vi "Differential_Yuhe.vi"(8 "dy/dx vs x":bool=TRUE, 9 "step":dbl=5.0, 10 "dv":dbl=5.0, 11 "A vs B":cluster{dbl[], dbl[]}[](graph)) -> (3 "A vs B 2":cluster{dbl[], dbl[]}[](graph))   [LabVIEW 2020]
uses:
  <vilib>/Analysis/baseanly.llb/Mean (DBL).vi
  <vilib>/Analysis/NI_AALPro.lvlib
  <vilib>/Analysis/NI_AALBase.lvlib
panel:
  in  "parameter bounds":T1={"amp min"=-inf, "amp max"=inf, "power min"=-inf, "power max"=inf, "offset min"=0.0, "offset max"=0.0}
  out "residue":dbl
  out "amplitude":dbl
  out "Fitoffset":dbl
  out "power":dbl
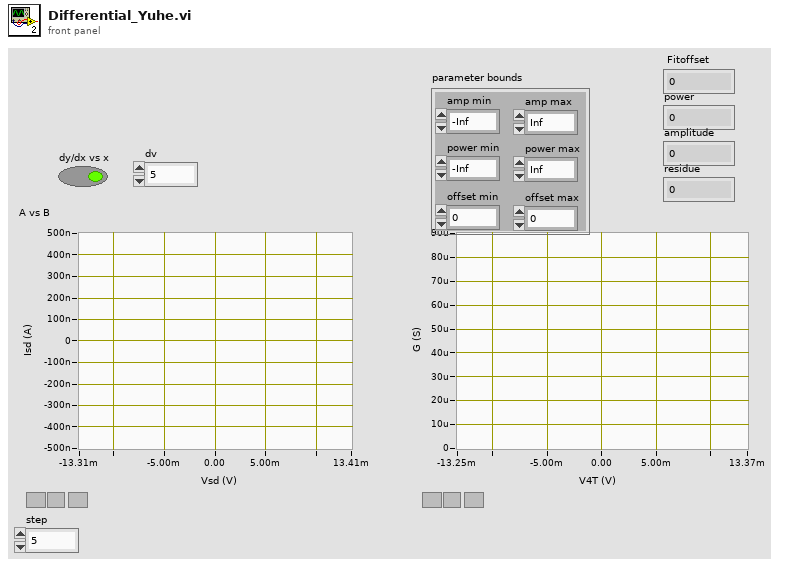
[diagram p1: front panel]
types:
  T1 = cluster{"amp min":dbl, "amp max":dbl, "power min":dbl, "power max":dbl, "offset min":dbl, "offset max":dbl}
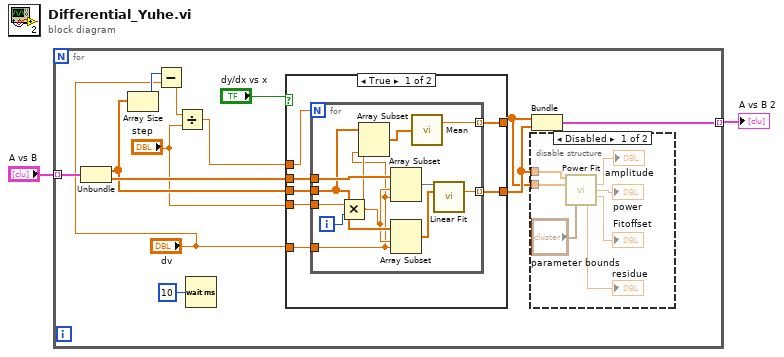
[diagram p0: block diagram]
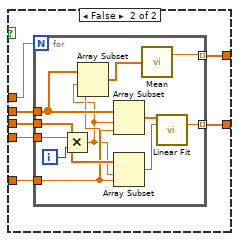
[diagram p3: hidden frame]
diagram:
  n1 = for {
    tunnel: "A vs B" -> [w13] mode=indexing
    tunnel: [w12] -> w1 mode=indexing
    n2 = Unbundle(w13) -> (w11:dbl[], w15:dbl[])
    n3 = Array Size(array=w11) -> (size(s)=w8:i32)
    n4 = Subtract(x=w8, y="dv") -> (x-y=w6:dbl)
    n5 = Divide(x=w6, y="step") -> (x/y=w10:dbl)
    n6 = Wait (ms)(milliseconds to wait=u32 10) -> ()  [unwired: 1 out]
    n7 = case shown="True" "dy/dx vs x" {
      tunnel: w10 -> [w29 w47]
      tunnel: "dv" -> [w28 w46]
      tunnel: [w27 w45] -> w4
      tunnel: w11 -> [w25 w43]
      tunnel: w15 -> [w26 w44]
      tunnel: [w23 w41] -> w3
      tunnel: "step" -> [w24 w42]
      frame True {
        n8 = for {
          N: w29 -> [_]
          tunnel: w25 -> [w34]
          tunnel: w26 -> [w40]
          tunnel: w28 -> [w32]
          tunnel: [w39] -> w27 mode=indexing
          tunnel: w24 -> [w38]
          tunnel: [w30] -> w23 mode=indexing
          i -> [w37]
          n9 = Multiply(x=w38, y=w37) -> (x*y=w33:dbl)
          n10 = Array Subset(array=w34, index=w33, length=w32) -> (w31:dbl[])
          n11 = Array Subset(array=w40, index=w33, length=w32) -> (w36:dbl[])
          n12 = Array Subset(array=w34, index=w33, length=w32) -> (w35:dbl[])
          n13 = call-poly <vilib>:"Mean.vi"("X"=w31) -> ("mean"=w30:dbl)  [unwired: 1 out]
          n14 = call <vilib>:"Linear Fit.vi"("Y"=w36, "X"=w35) -> ("slope"=w39:dbl)  [unwired: 9 in, 4 out]
        }
      }
      frame False {
        n15 = for {
          N: w47 -> [_]
          tunnel: w43 -> [w58]
          tunnel: w44 -> [w52]
          tunnel: w46 -> [w51]
          tunnel: [w57] -> w45 mode=indexing
          tunnel: w42 -> [w54]
          tunnel: [w48] -> w41 mode=indexing
          i -> [w53]
          n16 = Multiply(x=w54, y=w53) -> (x*y=w50:dbl)
          n17 = Array Subset(array=w52, index=w50, length=w51) -> (w49:dbl[])
          n18 = Array Subset(array=w52, index=w50, length=w51) -> (w56:dbl[])
          n19 = Array Subset(array=w58, index=w50, length=w51) -> (w55:dbl[])
          n20 = call-poly <vilib>:"Mean.vi"("X"=w49) -> ("mean"=w48:dbl)  [unwired: 1 out]
          n21 = call <vilib>:"Linear Fit.vi"("Y"=w56, "X"=w55) -> ("slope"=w57:dbl)  [unwired: 9 in, 4 out]
        }
      }
    }
    n22 = disable-structure shown="Disabled" {
      disable-tunnel: w4 -> [w18 _]
      disable-tunnel: w3 -> [w16 _]
      frame Disabled {
        n23 = call <vilib>:"Power Fit.vi"("Y"=w18, "X"=w16, "parameter bounds"="parameter bounds") -> ("amplitude"=→"amplitude":dbl, "power"=→"power":dbl, "offset"=→"Fitoffset":dbl, "residue"=→"residue":dbl)  [unwired: 7 in, 2 out]
      }
      frame Enabled {
      }
    }
    n24 = Bundle(w3, w4) -> (w12:cluster{dbl[], dbl[]})  [unwired: 1 in]
  }
  "A vs B 2" <- w1
